vi "buttonChange.vi"(8 "NC IN":bool, 11 "NO IN":bool) -> (0 "NO OUT":bool, 3 "NC OUT":bool)   [LabVIEW 2011]
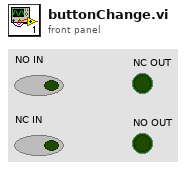
[diagram p1: front panel]
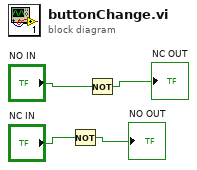
[diagram p0: block diagram]
diagram:
  n1 = Not(x="NC IN") -> (.not. x?=→"NO OUT":bool)
  n2 = Not(x="NO IN") -> (.not. x?=→"NC OUT":bool)
